vi "FrontalGalvoXYStand_Analog.vi"(8 "error in (no error)":errorcluster, 9 "stand Z vol backforth samp":cluster{"Fs":dbl, "#s":dbl}={"Fs"=500000.0, "#s"=200000.0}, 10 "Frontal Galvo xy scan range (V)":dbl=0.14 min=0.0 max=1.5, 11 "Frontal Galvo xy scan frequency (Hz)":i16=500 min=500 max=500) -> (0 "error out":errorcluster, 3 "FrontalGalvoXYStand":waveform(dbl))   [LabVIEW 2018]
uses:
  <vilib>/measure/NI_MABase.lvlib
panel:
  out "Preview":waveform(dbl)(graph)
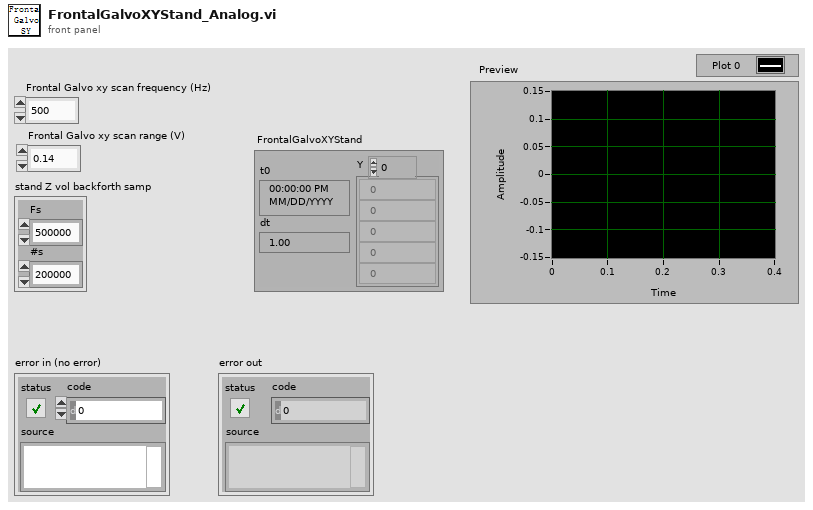
[diagram p1: front panel]
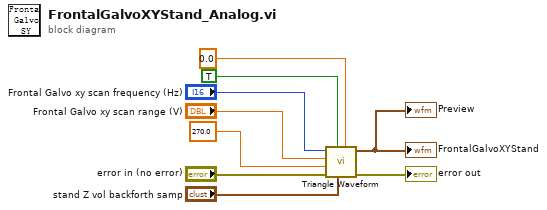
[diagram p0: block diagram]
diagram:
  n1 = call <vilib>:"Triangle Waveform.vi"("offset"=0.0, "sampling info"="stand Z vol backforth samp", "reset signal"=TRUE, "error in (no error)"="error in (no error)", "phase"=270.0, "amplitude"="Frontal Galvo xy scan range (V)", "frequency"="Frontal Galvo xy scan frequency (Hz)") -> ("error out"=→"error out":errorcluster, "signal out"=→"FrontalGalvoXYStand" →"Preview":waveform(dbl))  [unwired: 3 in]
